vi "3.1.1.-SubVI RGB a HSV.vi"(9 "B":u8, 10 "G":u8, 11 "R":u8) -> (1 "V":dbl, 2 "S":dbl, 3 "H":dbl)   [LabVIEW 2020]
doc: "Este subVI sirve para convertir un dato de color RGB a uno HSV"
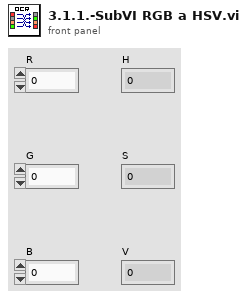
[diagram p1: front panel]
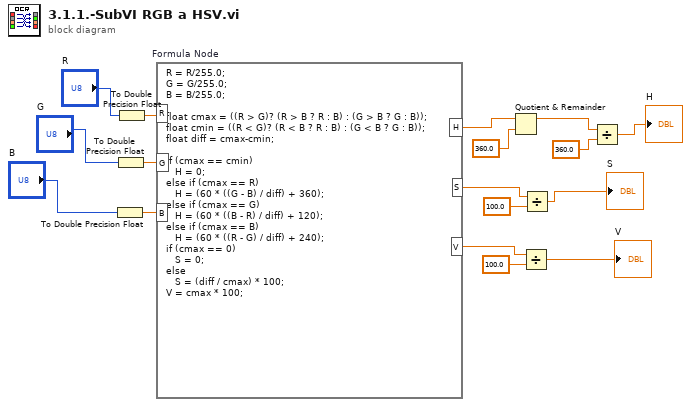
[diagram p0: block diagram]
diagram:
  n1 = To Double Precision Float(number="B") -> (double precision float=w6:dbl)
  n2 = To Double Precision Float(number="G") -> (double precision float=w3:dbl)
  n3 = To Double Precision Float(number="R") -> (double precision float=w2:dbl)
  n4 = formula code="R = R/255.0;\nG = G/255.0;\nB = B/255.0;\n\nfloat cmax = ((R > G)? (R > B ? R : B) : (G > B ? G : B));\nfloat cmin = ((R < G)? (R < B ? R : B) : (G < B ? G : B));\nfloat diff = cmax-cmin;\n\nif (cmax == cmin)\n   H = 0;\nelse if (cmax == R)\n   H = (60 * ((G - B) / diff) + 360);\nelse if (cmax == G)\n   H = (60 * ((B - R) / diff) + 120);\nelse if (cmax == B)\n   H = (60 * ((R - G) / diff) + 240);\nif (cmax == 0)\n   S = 0;\nelse\n   S = (diff / cmax) * 100;\nV = cmax * 100;"("R"=w2, "G"=w3, "B"=w6) -> ("H"=w8:dbl, "S"=w16:dbl, "V"=w17:dbl)
  n5 = Quotient & Remainder(x=w8, y=360.0) -> (x-y*floor(x/y)=w10:dbl)  [unwired: 1 out]
  n6 = Divide(x=w17, y=100.0) -> (x/y=→"V":dbl)
  n7 = Divide(x=w16, y=100.0) -> (x/y=→"S":dbl)
  n8 = Divide(x=w10, y=360.0) -> (x/y=→"H":dbl)
